vi "Status Set or Query SBR.vi"(0 "VISA resource name":refnum<visa-resource-name>, 5 "Set/Query (F:Query)":bool, 7 "Sent To Device (CH1-8 F:0)":T1, 11 "error in (no error)":errorcluster) -> (4 "VISA resource name out":refnum<visa-resource-name>, 8 "Read From Device":T1, 15 "error out":errorcluster)   [LabVIEW 2015, in "Chroma ATE 6310.lvlib"]
doc: "This VI sets or queries the bits in the instrument's IEEE-488.2 Status Byte register.\n\nWhen you choose \"Set\", you can use the control cluster \"Set To Instrument\" to set the register.And when choosing \"Query\", you can read status from the indicator cluster \"Read From Instrument\"."
uses:
  <instrlib>/Chroma ATE 6310/Chroma ATE 6310.lvlib
panel:
  # "Status Byte Register"
  # "Set\n\nQuery"
  # "-        MSS     ESB    MAV   QUES  CSUM      -           -\n   128       64        32        16          8          4          2          1"
  # "-        MSS     ESB    MAV   QUES  CSUM      -           -\n   128       64        32        16          8          4          2          1"
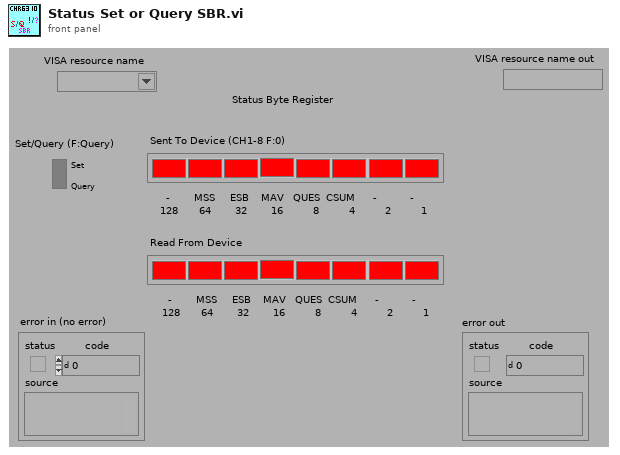
[diagram p1: front panel]
types:
  T1 = cluster{"Bit 7 (F:0)":bool, "Bit 6 (F:0)":bool, "Bit 5 (F:0)":bool, "Bit 4 (F:0)":bool, "Bit 3 (F:0)":bool, "Bit 2 (F:0)":bool, "Bit 1 (F:0)":bool, "Bit 0 (F:0)":bool}
  T2 = cluster{bool, bool, "Bit 5 (F:0)":bool, "Bit 4 (F:0)":bool, "Bit 3 (F:0)":bool, "Bit 2 (F:0)":bool, "Bit 1 (F:0)":bool, bool}
  T3 = cluster{bool, bool, bool, bool, bool, bool, bool, bool}
  T4 = cluster{"[0]":bool, "[1]":bool, "[2]":bool, "[3]":bool, "[4]":bool, "[5]":bool, "[6]":bool, "[7]":bool}
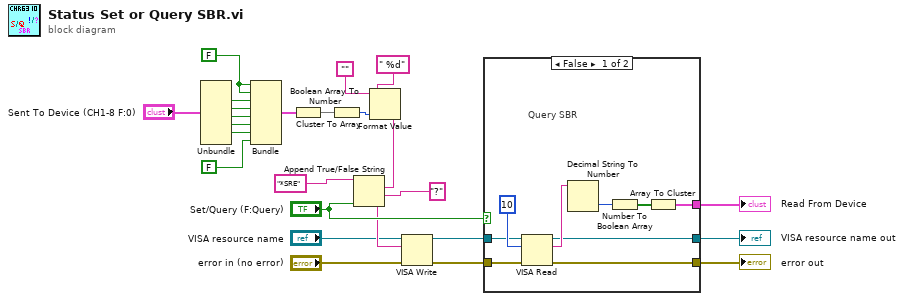
[diagram p0: block diagram]
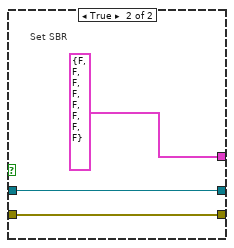
[diagram p2: hidden frame]
diagram:
  w11 = FALSE
  n1 = Unbundle("Sent To Device (CH1-8 F:0)") -> ("Bit 5 (F:0)"=w18:bool, "Bit 4 (F:0)"=w17:bool, "Bit 3 (F:0)"=w16:bool, "Bit 2 (F:0)"=w15:bool, "Bit 1 (F:0)"=w3:bool)  [unwired: 3 out]
  n2 = Bundle(w11, w11, "Bit 5 (F:0)"=w18, "Bit 4 (F:0)"=w17, "Bit 3 (F:0)"=w16, "Bit 2 (F:0)"=w15, "Bit 1 (F:0)"=w3, FALSE) -> (w4:T2)  [unwired: 1 in]
  n3 = Cluster To Array(cluster=w4) -> (array=w22:bool[])
  n4 = Boolean Array To Number(Boolean array=w22) -> (number=w21:u32)
  n5 = Format Value(string ("")="", format string=" %d", value (0)=w21) -> (output string=w24:string)
  n6 = Append True/False String(1:"Set/Query (F:Query)", 2:"?", 3:w24, 4:"*SRE") -> (0:w14:string)
  n7 = VISA Write(VISA resource name="VISA resource name", write buffer=w14, error in (no error)="error in (no error)") -> (VISA resource name out=w12:refnum<visa-resource-name>, error out=w13:errorcluster)  [unwired: 1 out]
  n8 = case shown="False" "Set/Query (F:Query)" {
    tunnel: w13 -> [w34 w37]
    tunnel: w12 -> [w29 w36]
    tunnel: [w28 w37] -> w7
    tunnel: [w27 w36] -> w6
    tunnel: [w26 T3 {FALSE, FALSE, FALSE, FALSE, FALSE, FALSE, FALSE, FALSE}] -> w1
    frame False {
      # "Query SBR"
      n9 = VISA Read(VISA resource name=w29, byte count=u32 10, error in (no error)=w34) -> (VISA resource name out=w27:refnum<visa-resource-name>, read buffer=w30:string, error out=w28:errorcluster)  [unwired: 1 out]
      n10 = Decimal String To Number(string=w30) -> (number=w33:i32)  [unwired: 2 in, 1 out]
      n11 = Number To Boolean Array(number=w33) -> (Boolean array=w32:bool[])
      n12 = Array To Cluster(array=w32) -> (cluster=w26:T4)
    }
    frame True {
      # "Set SBR"
    }
  }
  "error out" <- w7
  "VISA resource name out" <- w6
  "Read From Device" <- w1
